vi "10ms loop.vi"(6 "i":i32, 7 "Shooter Encoder":T2={"DevStatus"={"status"=FALSE, "code"=0, "source"=""}, "EncoderIndex"=enum."Invalid", "CounterIndex"=enum."Ctr 1", "DistancePerCount"=2.0, "Decoding Type"=enum."4x"}, 8 "Potent":T6, 9 "Arm Angle":T6, 10 "Shooter":T9, 11 "Driver":T9) -> ()   [LabVIEW 2012]
uses:
  <vilib>/Rock Robotics/WPI/AnalogChannel/WPI_AnalogChannelDevRef.ctl
  <vilib>/Rock Robotics/SystemInterfaces/Typedef/FPGA_TypedefAnalogModule.ctl
  <vilib>/Rock Robotics/SystemInterfaces/AI/FPGA_AIChannel.ctl
  <vilib>/Rock Robotics/WPI/Joystick/WPI_JoystickDevRef.ctl
  <vilib>/Rock Robotics/WPI/Joystick/WPI_JoystickDeviceEnum.ctl
  <vilib>/Rock Robotics/WPI/Encoder/WPI_EncoderDevRef.ctl
  <vilib>/Rock Robotics/SystemInterfaces/Encoder/FPGA_EncoderIdx.ctl
  <vilib>/Rock Robotics/SystemInterfaces/Counter/FPGA_CounterCtrSystemIndex.ctl
  <vilib>/Rock Robotics/WPI/Encoder/WPI_EncoderType.ctl
  Robot Global Data.vi
panel:
  out "Shooter":T1
  out "Loop Count":i32
  out "rps":dbl
  out "Arm Angle":dbl=1.71747033
  in  "Shooter":dbl=0.6
  out "Shooter (cps)":dbl
  out "Voltage":dbl=0.033620575
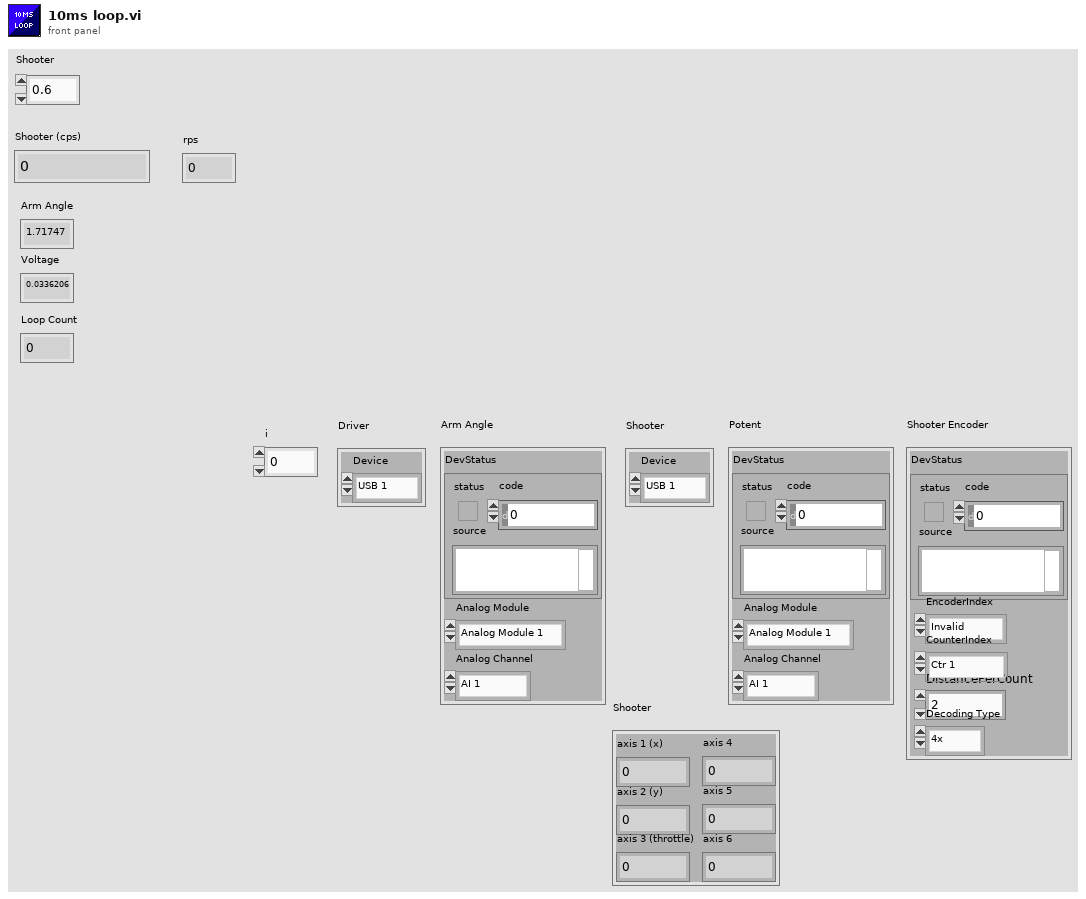
[diagram p1: front panel]
types:
  T1 = cluster{"axis 1 (x)":dbl, "axis 2 (y)":dbl, "axis 3 (throttle)":dbl, "axis 4":dbl, "axis 5":dbl, "axis 6":dbl}
  T2 = typedef "WPI_EncoderDevRef.ctl" = cluster{"DevStatus":errorcluster, "EncoderIndex":T3, "CounterIndex":T4, "DistancePerCount":dbl, "Decoding Type":T5}
  T3 = typedef "FPGA_EncoderIdx.ctl" = enum8{"Enc 0", "Enc 1", "Enc 2", "Enc 3", "Invalid"}
  T4 = typedef "FPGA_CounterCtrSystemIndex.ctl" = enum8{"Ctr 0", "Ctr 1", "Ctr 2", "Ctr 3", "Ctr 4", "Ctr 5", "Ctr 6", "Ctr 7", "Invalid"}
  T5 = typedef "WPI_EncoderType.ctl" = enum16{"1x", "2x", "4x"}
  T6 = typedef "WPI_AnalogChannelDevRef.ctl" = cluster{"DevStatus":errorcluster, "Analog Module":T7, "Analog Channel":T8}
  T7 = typedef "FPGA_TypedefAnalogModule.ctl" = enum16{"Analog Module 1", "Analog Module 2"}
  T8 = typedef "FPGA_AIChannel.ctl" = enum8{"AI 1", "AI 2", "AI 3", "AI 4", "AI 5", "AI 6", "AI 7", "AI 8", "Invalid"}
  T9 = typedef "WPI_JoystickDevRef.ctl" = cluster{"Device":T10}
  T10 = typedef "WPI_JoystickDeviceEnum.ctl" = enum16{"USB 1", "USB 2", "USB 3", "USB 4", "Kinect 1", "Kinect 2"}
  T11 = typedef "WPI_JoystickButtonState.ctl" = cluster{"Button 1":bool, "Button 2":bool, "Button 3":bool, "Button 4":bool, "Button 5":bool, "Button 6":bool, "Button 7":bool, "Button 8":bool, "Button 9":bool, "Button 10":bool, "Button 11":bool, "Button 12":bool}
  T12 = cluster{"Button 6":bool, "Button 7":bool, "Button 11":bool, "Button 10":bool, "Button 2":bool, "Button 3":bool, "Button 1":bool}
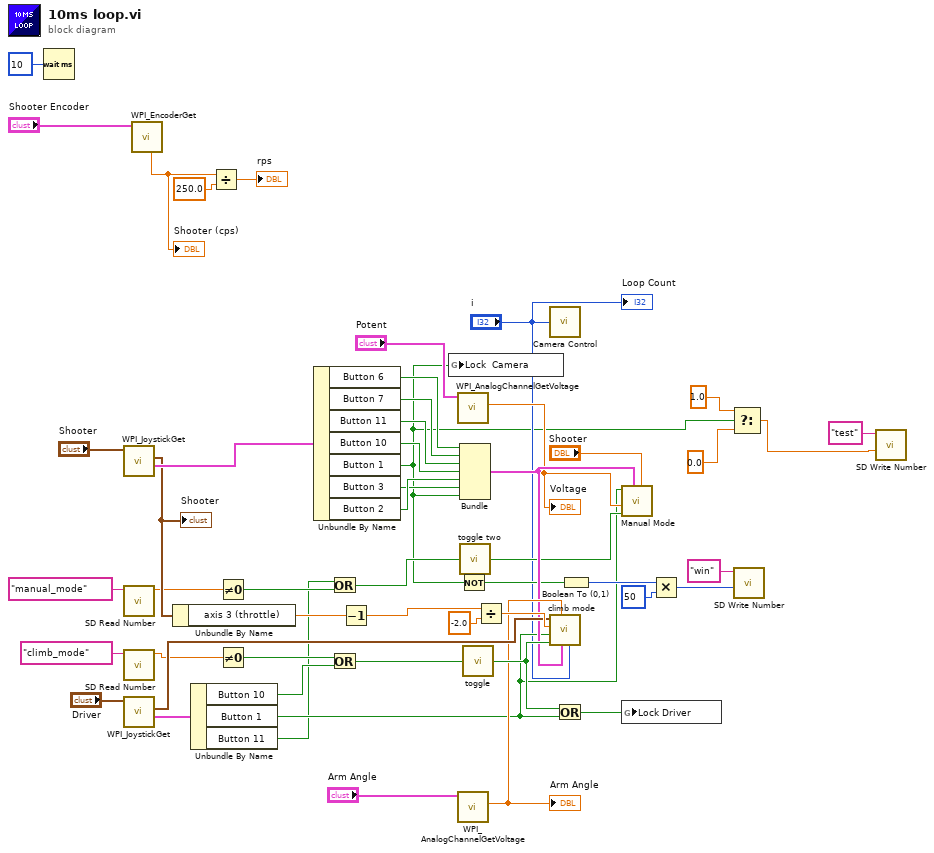
[diagram p0: block diagram]
diagram:
  n1 = Wait (ms)(milliseconds to wait=u32 10) -> ()  [unwired: 1 out]
  n2 = call <vilib>:"WPI_JoystickGet.vi"("JoystickDevRef"="Shooter") -> ("Buttons"=w50:T11, "Axes"=w44:T1)  [unwired: 4 in, 1 out]
  "Shooter" <- w44
  n3 = call <vilib>:"SD Read Number.vi"("Name"="manual_mode") -> ("Numeric"=w13:dbl)  [unwired: 8 in, 2 out]
  n4 = call <vilib>:"SD Read Number.vi"("Name"="climb_mode") -> ("Numeric"=w14:dbl)  [unwired: 8 in, 2 out]
  n5 = call <vilib>:"WPI_JoystickGet.vi"("JoystickDevRef"="Driver") -> ("Buttons"=w51:T11, "Axes"=w33:T1)  [unwired: 4 in, 1 out]
  n6 = call <vilib>:"WPI_EncoderGet.vi"("EncoderDevRef"="Shooter Encoder") -> ("Rate"=w38:dbl)  [unwired: 5 in, 5 out]
  "Shooter (cps)" <- w38
  n7 = Unbundle By Name(w44) -> ("axis 3 (throttle)"=w41:dbl)
  n8 = Unbundle By Name(w51) -> ("Button 10"=w10:bool, "Button 1"=w22:bool, "Button 11"=w7:bool)
  n9 = Divide(x=w38, y=250.0) -> (x/y=→"rps":dbl)
  n10 = Not Equal To 0?(x=w13) -> (x != 0?=w8:bool)
  n11 = Not Equal To 0?(x=w14) -> (x != 0?=w15:bool)
  n12 = Unbundle By Name(w50) -> ("Button 6"=w48:bool, "Button 7"=w47:bool, "Button 11"=w46:bool, "Button 10"=w45:bool, "Button 1"=w4:bool, "Button 3"=w39:bool, "Button 2"=w40:bool)
  n13 = Or(x=w7, y=w8) -> (x .or. y?=w6:bool)
  n14 = Or(x=w15, y=w10) -> (x .or. y?=w9:bool)
  n15 = Decrement(x=w41) -> (x-1=w42:dbl)
  n16 = global write "Robot Global Data.vi" "Lock  Camera"(w4) -> ()
  n17 = call <vilib>:"WPI_AnalogChannelGetVoltage.vi"("AIDeviceRef"="Potent") -> ("Voltage"=w29:dbl)  [unwired: 8 in, 2 out]
  "Voltage" <- w29
  n18 = call <vilib>:"WPI_AnalogChannelGetVoltage.vi"("AIDeviceRef"="Arm Angle") -> ("Voltage"=w32:dbl)  [unwired: 8 in, 2 out]
  "Arm Angle" <- w32
  n19 = Not(x=w4) -> (.not. x?=w23:bool)
  n20 = Bundle("Button 6"=w48, "Button 7"=w47, "Button 11"=w46, "Button 10"=w45, "Button 2"=w40, "Button 3"=w39, "Button 1"=w4) -> (w30:T12)  [unwired: 1 in]
  n21 = call "toggle two.vi"("Button In"=w6) -> ("tggle Out"=w25:bool)
  n22 = call "toggle.vi"("Btn In"=w9) -> ("Toggle Out"=w35:bool)
  n23 = Divide(x=w42, y=-2.0) -> (x/y=w34:dbl)
  n24 = call "Camera Control.vi"("i"="i") -> ()  [unwired: 1 in]
  n25 = call "climb mode.vi"("i"="i", "Joystick 2"=w30, "Arm Angle"=w32, "engage climb"=w35, "Button 1"=w22, "Slide"=w34, "Joystick 1 Axes"=w33) -> ()  [unwired: 5 in]
  n26 = Or(x=w35, y=w22) -> (x .or. y?=w49:bool)
  n27 = Boolean To (0,1)(Boolean=w23) -> (0, 1=w28:i16)
  n28 = call "Manual Mode.vi"("slider shoot"="Shooter", "Shooter"=w30, "engage shoot"=w25, "Potent"=w29, "Button 1"=w22) -> ()  [unwired: 7 in]
  n29 = global write "Robot Global Data.vi" "Lock Driver"(w49) -> ()
  n30 = Multiply(x=w28, y=i16 50) -> (x*y=w27:i16)
  n31 = Select(t=1.0, s=w4, f=0.0) -> (s? t:f=w3:dbl)
  n32 = call <vilib>:"SD Write Number.vi"("Numeric"=w27, "Name"="win") -> ()  [unwired: 8 in, 2 out]
  n33 = call <vilib>:"SD Write Number.vi"("Numeric"=w3, "Name"="test") -> ()  [unwired: 8 in, 2 out]
  "Loop Count" <- "i"
